vi "总时间.vi"(8 "已运行时间 2":refnum<vi>, 9 "剩余时间 2":refnum<vi>, 10 "设定运行时间 2":refnum<vi>, 11 "millisecond timer value":u32) -> ()   [LabVIEW 2012]
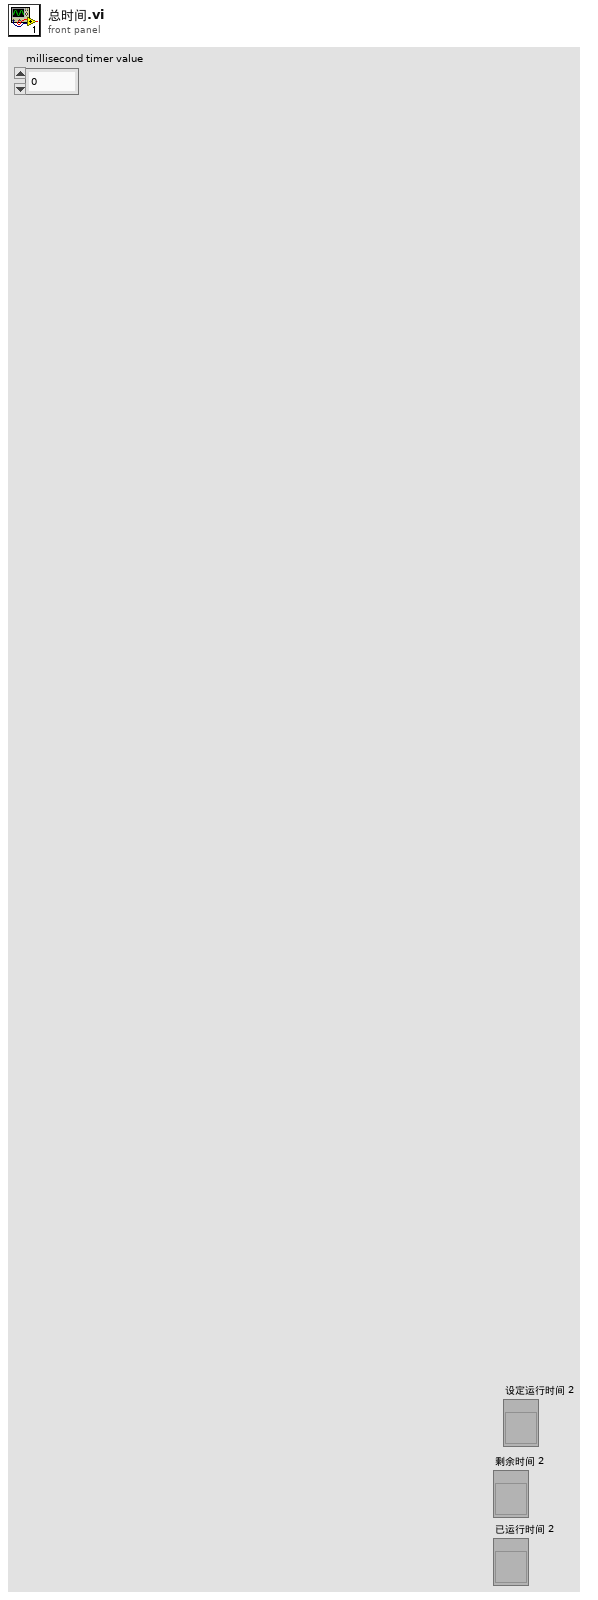
[diagram p1: front panel]
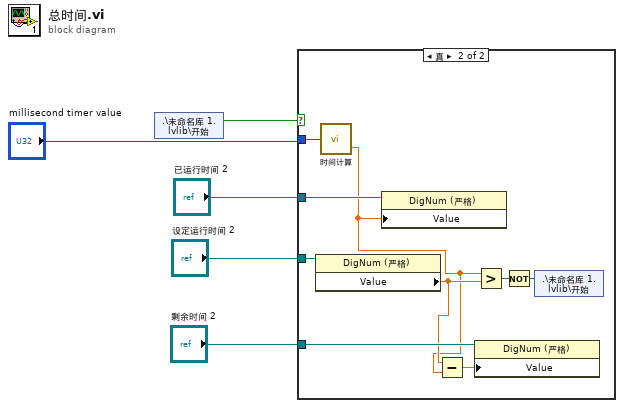
[diagram p0: block diagram]
diagram:
  n1 = shared-variable ".\\未命名库 1.lvlib\\开始"() -> (w4:bool)  [unwired: 1 in, 1 out]
  n2 = case shown="真" w4 {
    tunnel: "millisecond timer value" -> [_ w14]
    tunnel: "已运行时间 2" -> [_ w13]
    tunnel: "剩余时间 2" -> [_ w12]
    tunnel: "设定运行时间 2" -> [_ w11]
    frame False {
    }
    frame True {
      n3 = property class="DigNum (严格)"(reference=w11) -> ("Value"=w7:dbl)  [unwired: 1 in, 2 out]
      n4 = call "时间计算.vi"("跳变时间"=w14) -> ("数值"=w6:dbl)  [unwired: 1 out]
      n5 = property class="DigNum (严格)"(reference=w13, "Value"=w6) -> ()  [unwired: 1 in, 2 out]
      n6 = Subtract(x=w7, y=w6) -> (x-y=w8:dbl)
      n7 = property class="DigNum (严格)"(reference=w12, "Value"=w8) -> ()  [unwired: 1 in, 2 out]
      n8 = Greater?(x=w6, y=w7) -> (0:w10:bool)
      n9 = Not(x=w10) -> (.not. x?=w9:bool)
      n10 = shared-variable ".\\未命名库 1.lvlib\\开始"(w9) -> ()  [unwired: 1 in, 1 out]
    }
  }
